vi "cDAQ Get AI Data.vi"(8 "Error In":errorcluster, 11 "Input Task":refnum<k21>) -> (0 "Error Out":errorcluster, 2 "Mean & StdDev":T1[](array[typedef]), 3 "Task Out":refnum<k21>, 5 "Measurements":dbl[][](array[numeric]) format="%0.2f")   [LabVIEW 2016]
doc: "Read analog input voltages through NI Max. Configurations for NI Max are listed on block diagram."
uses:
  <vilib>/Analysis/NI_AALBase.lvlib
  <vilib>/DAQmx/read.llb/DAQmx Read (Analog 2D DBL NChan NSamp).vi
  Type Definitions/Instrument Sensor.ctl
panel:
  out "Voltages Graph":dbl[][](graph)
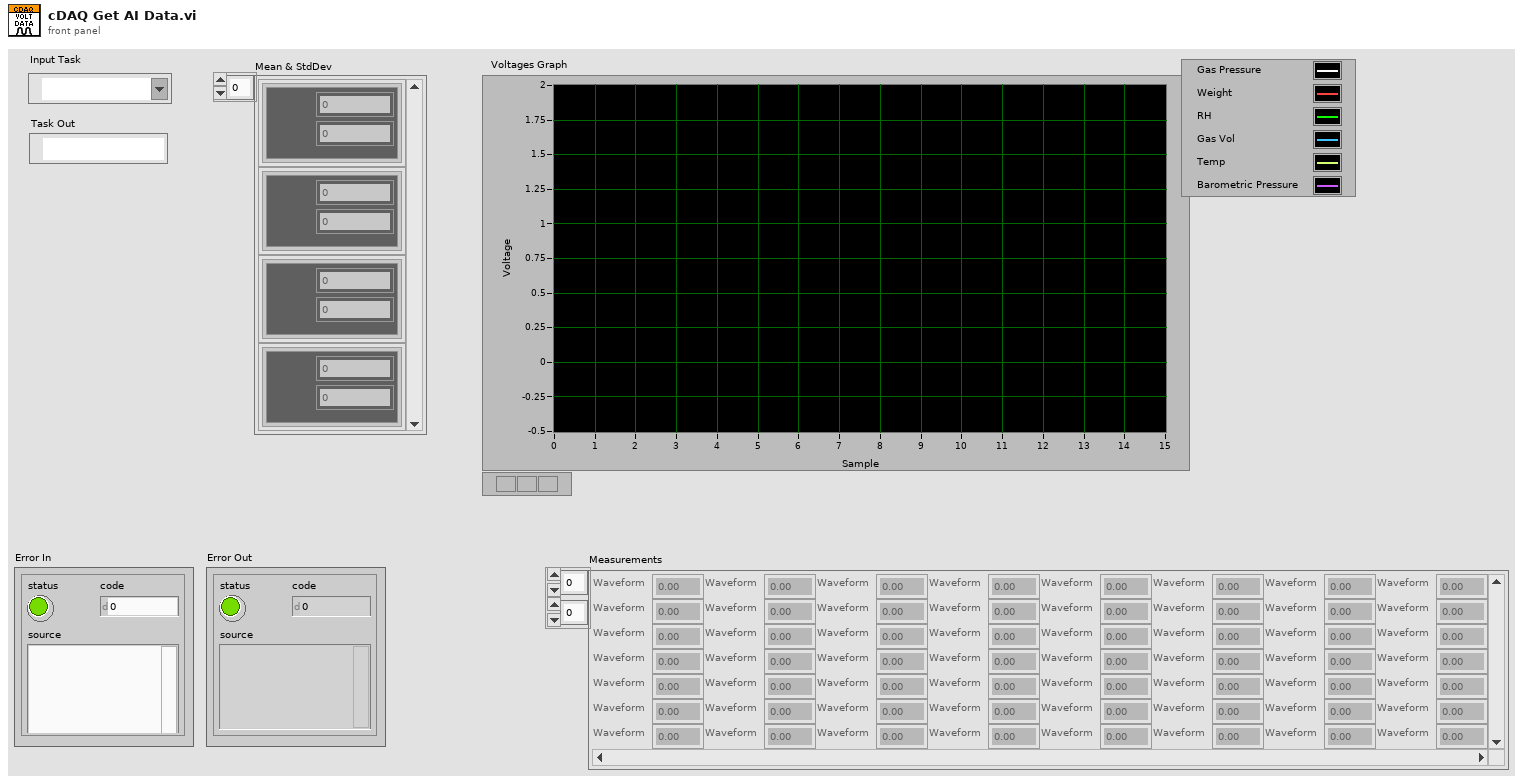
[diagram p1: front panel]
types:
  T1 = typedef "Instrument Sensor.ctl" = cluster{"Mean":dbl, " Std":dbl, "Color Box":u32}
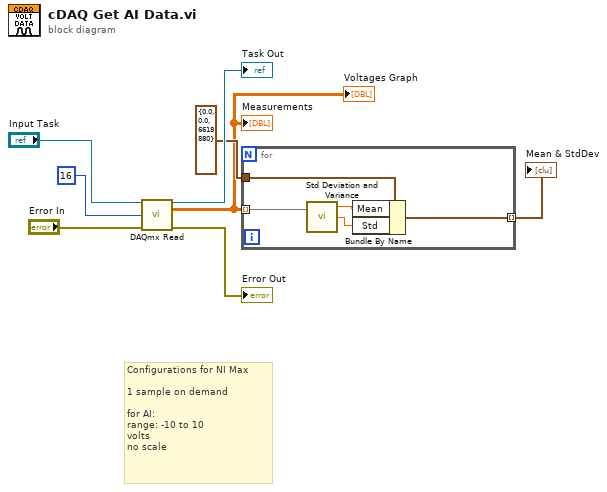
[diagram p0: block diagram]
diagram:
  # "Configurations for NI Max\n\n1 sample on demand \n\nfor AI: \nrange: -10 to 10 \nvolts\nno scale"
  n1 = call-poly <vilib>:"DAQmx Read.vi"("task/channels in"="Input Task", "number of samples per channel"=16, "error in"="Error In") -> ("task out"=→"Task Out":refnum<k21>, "data"=w1:dbl[][], "error out"=→"Error Out":errorcluster)  [unwired: 10 in]
  "Measurements" <- w1
  "Voltages Graph" <- w1
  n2 = for {
    tunnel: w1 -> [w13] mode=indexing
    tunnel: [w10] -> w2 mode=indexing
    tunnel: T1 {"Mean"=0.0, " Std"=0.0, "Color Box"=6618880} ("cluster") -> [w9]
    n3 = call <vilib>:"Std Deviation and Variance.vi"("X"=w13) -> ("mean"=w12:dbl, "standard deviation"=w11:dbl)  [unwired: 1 in, 1 out]
    n4 = Bundle By Name(cluster=w9, "Mean"=w12, "Std"=w11) -> (w10:T1)
  }
  "Mean & StdDev" <- w2
